vi "$CNXN_MC18V7.vi"() -> ()   [LabVIEW 2024]
panel:
  in  "Send":bool
  out "error out":errorcluster
  out "Connected":bool
  out "read buffer":string
  in  "Tx Buf Out":string
  in  "stop":bool
  # "0xC2 is the \"get firmware Version command\"\nShould return 0xA100 0401.\nBe sure buffers are in HEX display mode."
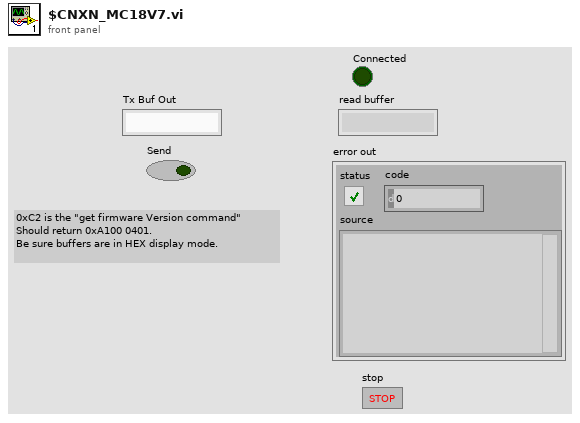
[diagram p1: front panel]
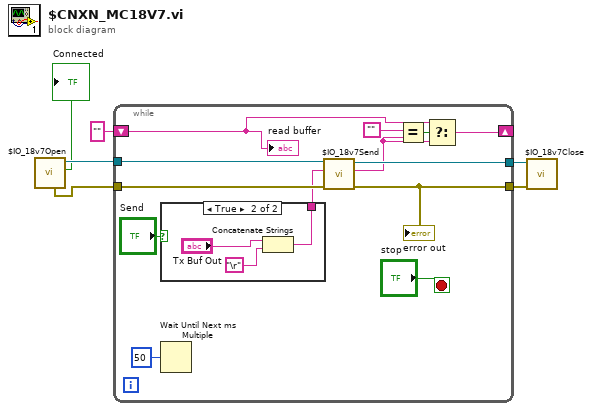
[diagram p0: block diagram]
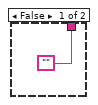
[diagram p2: hidden frame]
diagram:
  n1 = call "$IO_18v7Open.vi"() -> ("Connected"=→"Connected":bool, "VISA Refnum out"=w6:refnum<visa-resource-name>, "error out"=w4:errorcluster)  [unwired: 9 in]
  n2 = while {
    tunnel: w6 -> [w18]
    tunnel: [w17] -> w5
    tunnel: w4 -> [w16]
    tunnel: [w15] -> w3
    shift-right: [w9] -> _
    shift-left: "" ("read buffer") -> [w7]
    stop <- "stop" stop-if-true
    n3 = case shown="True" "Send" {
      tunnel: ["" w23] -> w14
      frame False {
      }
      frame True {
        n4 = Concatenate Strings("Tx Buf Out", "\r") -> (w23:string)
      }
    }
    n5 = Wait Until Next ms Multiple(millisecond multiple=u32 50) -> ()  [unwired: 1 out]
    n6 = call "$IO_18v7Send.vi"("error in (no error)"=w16, "Tx Buf Out"=w14, "VISA Refnum in"=w18) -> ("error out"=w15:errorcluster, "read buffer"=w10:string, "VISA Refnum out"=w17:refnum<visa-resource-name>)  [unwired: 6 in]
    "error out" <- w15
    n7 = Equal?(x="", y=w10) -> (x = y?=w11:bool)
    n8 = Select(t=w7, s=w11, f=w10) -> (s? t:f=w9:string)
    "read buffer" <- w7
  }
  n9 = call "$IO_18v7Close.vi"("error in (no error)"=w3, "VISA Refnum in"=w5) -> ()  [unwired: 10 in]
